vi "FT to Encoder Ticks.vi"(11 "Ft":dbl) -> (3 "Ticks":dbl)   [LabVIEW 2017]
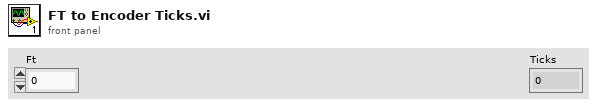
[diagram p1: front panel]
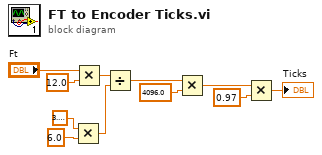
[diagram p0: block diagram]
diagram:
  n1 = Multiply(x=3.141592653589793, y=6.0) -> (x*y=w6:dbl)
  n2 = Multiply(x="Ft", y=12.0) -> (x*y=w4:dbl)
  n3 = Divide(x=w4, y=w6) -> (x/y=w5:dbl)
  n4 = Multiply(x=w5, y=4096.0) -> (x*y=w10:dbl)
  n5 = Multiply(x=w10, y=0.97) -> (x*y=→"Ticks":dbl)
